vi "System Curve Name Replace.vi"(8 "Hardware in":string, 9 "Step Setup in":string, 10 "Setup in":T1={"No.VI"=0, "Category"="", "StepName"="", "Seq setup flattened"="", "Comment"="", "Steps config."=[], "Jump config"=[], "Start"=0.0, "Increment"=0.0, "Name"="Pa", "Unit"="Pa", "Y data"=1, "Y prefix"="", "Y dB ref"=1.0, "Y unit"="", "Repeat State Array"=[]} {"Repeat State Array"."Start" format="%#_5g"; "Y dB ref" format="%.1f"; "Y data" items=["dB", "Lin"]; "Start" format="%#_5g"}, 11 "Type In":string) -> (3 "Inserted Names Out":string[](array[string]))   [LabVIEW 2013]
uses:
  CRYCustom and Run Seq.llb/CRYStep.ctl
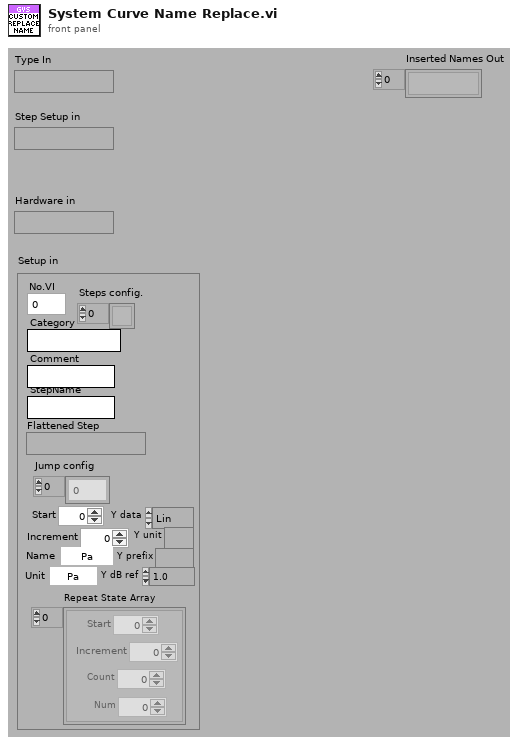
[diagram p1: front panel]
types:
  T1 = typedef "CRYStep.ctl" = cluster{"No.VI":i32, "Category":string, "StepName":string, "Seq setup flattened":string, "Comment":string, "Steps config.":bool[], "Jump config":i32[], "Start":dbl, "Increment":dbl, "Name":string, "Unit":string, "Y data":u16, "Y prefix":string, "Y dB ref":dbl, "Y unit":string, "Repeat State Array":cluster{"Start":dbl, "Increment":dbl, "Count":i32, "Num":i32}[]}
  T2 = cluster{"Command Line":string, "Working Directory":path, "WaitForCompletion":bool}
  T3 = typedef "CRYCustom Cluster.ctl" = cluster{"Help":string, "Flatten Data":string}
  T4 = typedef "CRYData Cluster.ctl" = cluster{"Name":string, "Curve":cluster{"x":dbl, "y":dbl, "z":dbl}[], "X data":u16, "Y data":u16, "Z data":u16, "X axis":u16, "Y axis":u16, "Z axis":u16, "X unit":string, "Y unit":string, "Z unit":string, "X dB ref":dbl, "Y dB ref":dbl, "Z dB ref":dbl, "single val":bool, "protected":bool, "display X":bool, "display Y":bool, "display Z":bool, "Test Info":string, "Step No.":i32, "Plot Settings":cluster{"Color":u32, "Interpolation":u8, "Point Style":u8, "Line Style":u8, "Point Color":u32, "Line Width":u8, "Bar Plot Style":u8, "Fill To":i16}, "AutoProtect":bool}
  T5 = typedef "CRYWaveform Cluster.ctl" = cluster{"Waveform":cluster{"X0":dbl, "dX":dbl, "Y":sgl[]}, "X data":u16, "Y data":u16, "Y axis":u16, "X unit":string, "Y unit":string, "Y dB ref":dbl, "display Y":bool, "display X":bool, "Overload?":bool, "Test Info":string, "Step No.":i32, "Name":string, "protected":bool, "Sqc history":string[], "Signal Channel ID":i32, "Plot Settings":cluster{"Color":u32, "Interpolation":u8, "Point Style":u8, "Line Style":u8, "Point Color":u32, "Line Width":u8, "Bar Plot Style":u8, "Fill To":i16}, "AutoProtect":bool}
  T6 = typedef "CRYResult Cluster.ctl" = cluster{"Name":string, "Margin":dbl, "unit":string, "Verdict":bool, "Limit":string, "Max/Min":string, "protected":bool, "Step No.":i32, "Test Info":string, "AutoProtect":bool}
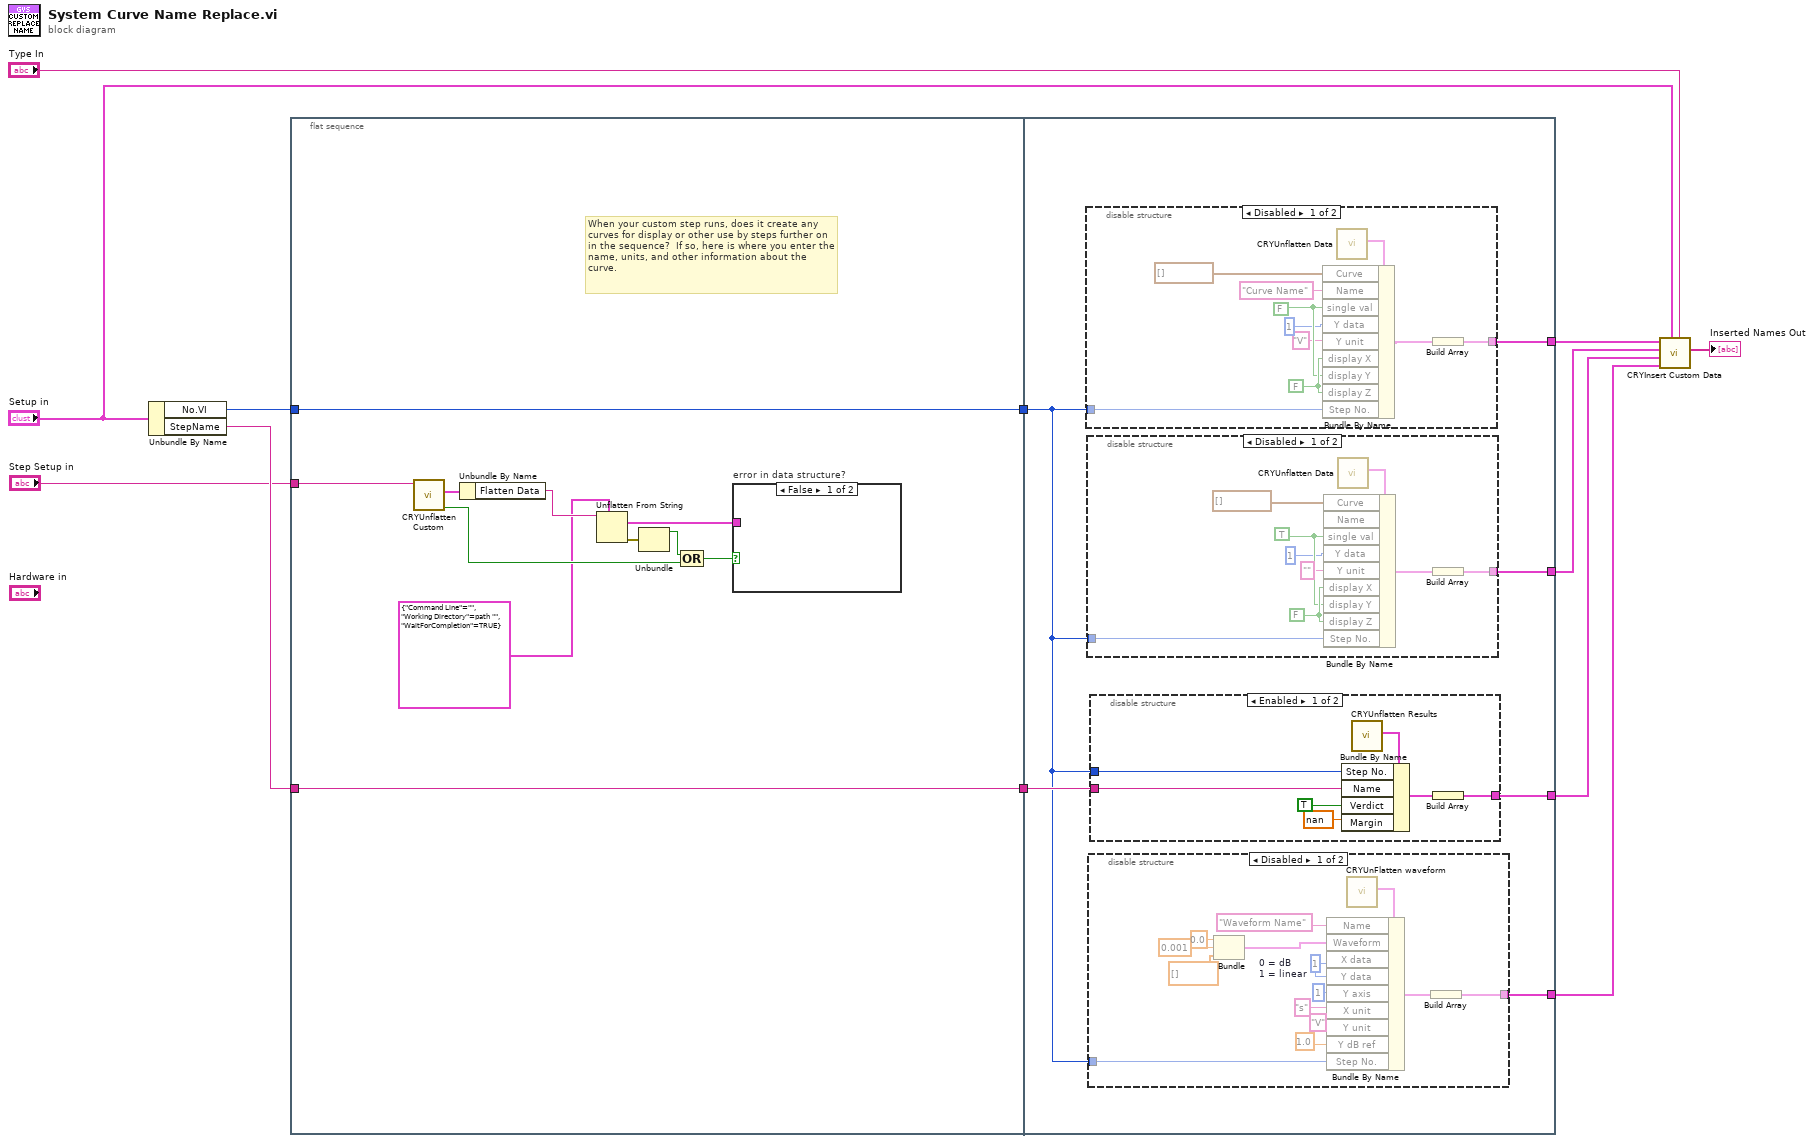
[diagram p0: block diagram]
diagram:
  n1 = Unbundle By Name("Setup in") -> ("No.VI"=w9:i32, "StepName"=w10:string)
  n2 = flat-sequence {
    tunnel: w9 -> [w22]
    tunnel: w10 -> [w23]
    tunnel: [w23] -> w4
    tunnel: [w22] -> w3
    tunnel: "Step Setup in" -> [w14]
    tunnel: [w27] -> w8
    tunnel: [w26] -> w6
    tunnel: [w25] -> w5
    tunnel: [w24] -> w7
    tunnel: w4 -> [w29]
    tunnel: w3 -> [w28]
    frame #0 {
      # "When your custom step runs, does it create any curves for display or other use by steps further on in the sequence?  If so, here is where you enter the name, units, and other information about the curve."
      n3 = call "CRYUnflatten Custom.vi"("Unflatten Custom"=w14) -> ("Error?"=w15:bool, "Custom"=w17:T3)  [unwired: 8 in, 1 out]
      n4 = Unbundle By Name(w17) -> ("Flatten Data"=w16:string)
      n5 = Unflatten From String(type=T2 {"Command Line"="", "Working Directory"=path "", "WaitForCompletion"=TRUE}, binary string=w16) -> (value=w20:T2, error out=w21:errorcluster)  [unwired: 1 in, 3 out]
      n6 = Unbundle(w21) -> ("status"=w18:bool)  [unwired: 2 out]
      n7 = Compound Arithmetic op=OR(w18, w15) -> (w19:bool)
      n8 = case "error in data structure?" shown="False" w19 {
        tunnel: w20 -> [_ _]
        frame False {
        }
        frame True {
        }
      }
    }
    frame #1 {
      n9 = disable-structure shown="Disabled" {
        disable-tunnel: w28 -> [w35 _]
        disable-tunnel: [w30 _] -> w27
        frame Disabled {
          w38 = FALSE
          w37 = FALSE
          n10 = call "CRYUnflatten Data.vi"() -> ("Datum"=w39:T4)  [unwired: 9 in, 2 out]
          n11 = Bundle By Name(cluster=w39, "Curve"=cluster{"x":dbl, "y":dbl, "z":dbl}[] [] ("appended array"), "Name"="Curve Name", "single val"=w37, "Y data"=u16 1, "Y unit"="V", "display X"=w38, "display Y"=w37, "display Z"=w38, "Step No."=w35) -> (w31:T4)
          n12 = Build Array(w31) -> (w30:T4[])
        }
        frame Enabled {
        }
      }
      n13 = disable-structure shown="Disabled" {
        disable-tunnel: w28 -> [w44 _]
        disable-tunnel: [w42 _] -> w24
        frame Disabled {
          w47 = FALSE
          w46 = TRUE
          n14 = call "CRYUnflatten Data.vi"() -> ("Datum"=w48:T4)  [unwired: 9 in, 2 out]
          n15 = Bundle By Name(cluster=w48, "Curve"=cluster{"x":dbl, "y":dbl, "z":dbl}[] [] ("appended array"), "single val"=w46, "Y data"=u16 1, "Y unit"="", "display X"=w47, "display Y"=w46, "display Z"=w47, "Step No."=w44) -> (w43:T4)  [unwired: 1 in]
          n16 = Build Array(w43) -> (w42:T4[])
        }
        frame Enabled {
        }
      }
      n17 = disable-structure shown="Disabled" {
        disable-tunnel: [w57 _] -> w25
        disable-tunnel: w28 -> [w56 _]
        frame Disabled {
          w62 = u16 1  # 0 = dB 1 = linear
          n18 = Bundle ("Actual waveform data bundle.\nX0\ndX\n[Y] array")(0.0, 0.001, dbl[] []) -> (w66:cluster{dbl, dbl, dbl[]})  [unwired: 1 out]
          n19 = call "CRYUnFlatten waveform.vi"() -> ("Waveform Cluster"=w67:T5)  [unwired: 9 in, 2 out]
          n20 = Bundle By Name(cluster=w67, "Name"="Waveform Name" ("Bundle Element"), "Waveform"=w66, "X data"=w62, "Y data"=w62, "Y axis"=u16 1, "X unit"="s", "Y unit"="V", "Y dB ref"=1.0, "Step No."=w56) -> (w68:T5)
          n21 = Build Array(w68) -> (w57:T5[])
        }
        frame Enabled {
        }
      }
      n22 = disable-structure shown="Enabled" {
        disable-tunnel: w28 -> [w51 _]
        disable-tunnel: w29 -> [w50 _]
        disable-tunnel: [w49 _] -> w26
        frame Enabled {
          n23 = call "CRYUnflatten Results.vi"() -> ("Result"=w52:T6)  [unwired: 9 in, 2 out]
          n24 = Bundle By Name(cluster=w52, "Step No."=w51, "Name"=w50, "Verdict"=TRUE, "Margin"=nan) -> (w54:T6)
          n25 = Build Array(w54) -> (w49:T6[])
        }
        frame Disabled {
        }
      }
    }
  }
  n26 = call "CRYInsert Custom Data.vi"("sAction"="Type In", "Setup in"="Setup in", "Wave"=w5, "Results"=w6, "Values"=w7, "Curves"=w8) -> ("Inserted Names Out"=→"Inserted Names Out":string[])  [unwired: 4 in, 1 out]
